vi "Example Cluster Bundler and Shift Register.vi"() -> ()   [LabVIEW 2018]
uses:
  Example Translator Vis/Example Vector of Floats.ctl
panel:
  out "Cluster 2":T1
  out "Cluster":T1
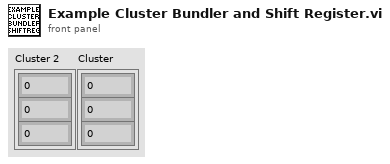
[diagram p1: front panel]
types:
  T1 = typedef "Example Vector of Floats.ctl" = cluster{sgl, sgl, sgl}
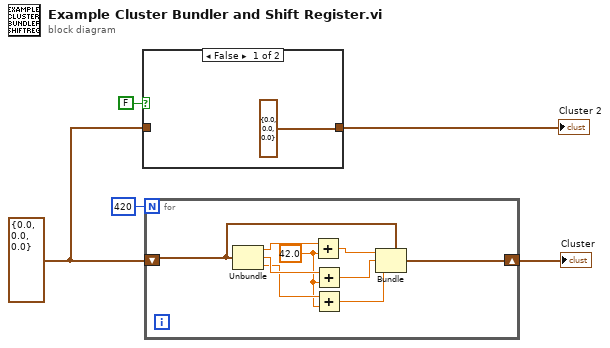
[diagram p0: block diagram]
diagram:
  w3 = T1 {0.0, 0.0, 0.0}
  n1 = case shown="False" FALSE {
    tunnel: w3 -> [_ w7]
    tunnel: [cluster{sgl, sgl, sgl} {0.0, 0.0, 0.0} w7] -> w1
    frame False {
    }
    frame True {
    }
  }
  "Cluster 2" <- w1
  n2 = for {
    N: 420 -> [_]
    shift-right: [w8] -> w4
    shift-left: w3 -> [w16]
    w12 = sgl 42.0 ("y")
    n3 = Unbundle(w16) -> (w15:sgl, w14:sgl, w13:sgl)
    n4 = Add(x=w15, y=w12) -> (x+y=w11:sgl)
    n5 = Add(x=w14, y=w12) -> (x+y=w10:sgl)
    n6 = Add(x=w13, y=w12) -> (x+y=w9:sgl)
    n7 = Bundle(cluster=w16, w11, w10, w9) -> (w8:T1)
  }
  "Cluster" <- w4
